vi "Query Command.vi"(0 "RedPitaya connection in":refnum<k5>, 2 "Query setting":u16(ring) items=["State of Digital IOs", "Analog Voltage", "Decimation", "Sampling Rate", "Sampling Rate (Hz)", "Averaging Status", "Trigger Status", "Trigger Delay in Samples", "Trigger Delay in ns", "Trigger Level in mV", "Current Position of Write Pointer", "Position of Trigger Event", "Buffer Size"], 3 "Pin Name":string, 5 "error in":errorcluster, 12 "timeout ms (2000)":i32=2000) -> (14 "RedPitaya connection out":refnum<k5>, 16 "Output string":string, 19 "error out":errorcluster)   [LabVIEW 2021, in "RedPitaya.lvlib"]
doc: "Returns specific information from Red Pitaya. If the query is about a specific pin, you have to provide the pin ID to <b>Pin Name</b> using one of the following descriptors DIO1 _P...DIO7_P, DIO0_N...DIO7_N."
uses:
  RedPitaya.lvlib
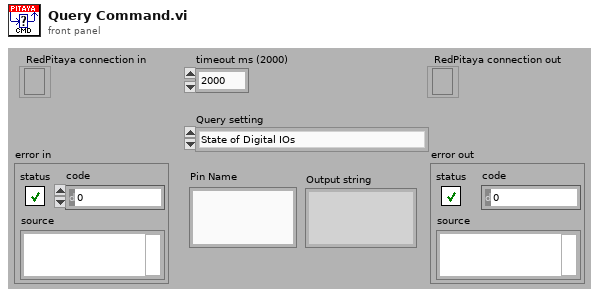
[diagram p1: front panel]
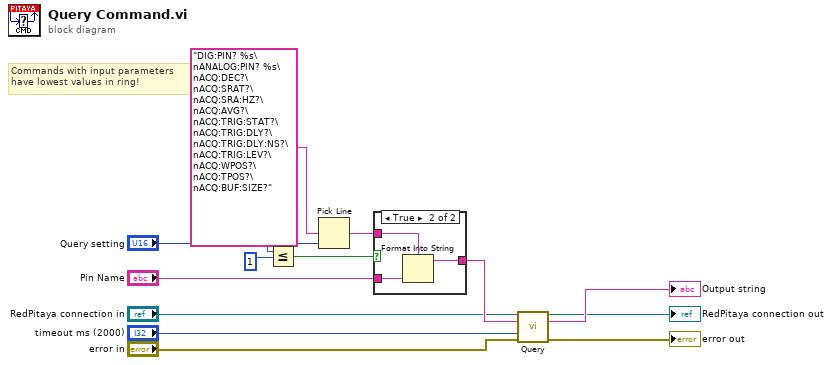
[diagram p0: block diagram]
diagram:
  # "Commands with input parameters\nhave lowest values in ring!"
  n1 = Less Or Equal?(x="Query setting", y=u16 1) -> (x <= y?=w10:bool)
  n2 = Pick Line(multi-line string="DIG:PIN? %s\nANALOG:PIN? %s\nACQ:DEC?\nACQ:SRAT?\nACQ:SRA:HZ?\nACQ:AVG?\nACQ:TRIG:STAT?\nACQ:TRIG:DLY?\nACQ:TRIG:DLY:NS?\nACQ:TRIG:LEV?\nACQ:WPOS?\nACQ:TPOS?\nACQ:BUF:SIZE?", line index="Query setting") -> (output string=w7:string)  [unwired: 1 in]
  n3 = case shown="True" w10 {
    tunnel: [w14 w17] -> w11
    tunnel: "Pin Name" -> [_ w16]
    tunnel: w7 -> [w14 w15]
    frame False {
    }
    frame True {
      n4 = Format Into String(format string=w15, w16) -> (resulting string=w17:string)  [unwired: 2 in, 1 out]
    }
  }
  n5 = call "Query.vi"("RedPitaya connection in"="RedPitaya connection in", "SCPI Query"=w11, "timeout ms (2000)"="timeout ms (2000)", "error in"="error in") -> ("RedPitaya connection out"=→"RedPitaya connection out":refnum<k5>, "data out"=→"Output string":string, "error out"=→"error out":errorcluster)  [unwired: 9 in]
